vi "Read states.vi"(8 "error in (no error)":errorcluster, 11 "NewTestTactic in":refnum<class "NewTestTactic.lvclass">) -> (0 "error out":errorcluster, 2 "states":T1, 3 "NewTestTactic out":refnum<class "NewTestTactic.lvclass">)   [LabVIEW 2022 SP3, in "NewTestTactic.lvclass"]
uses:
  NewTestTactic.lvclass
  Control 1.ctl
  NewTestTactic.lvclass/NewTestTactic.ctl
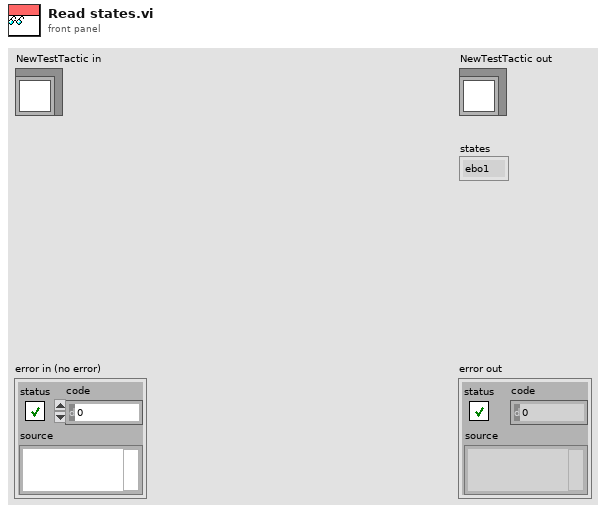
[diagram p1: front panel]
types:
  T1 = typedef "Control 1.ctl" = enum16{"ebo1", "ebo2", "bo3"}
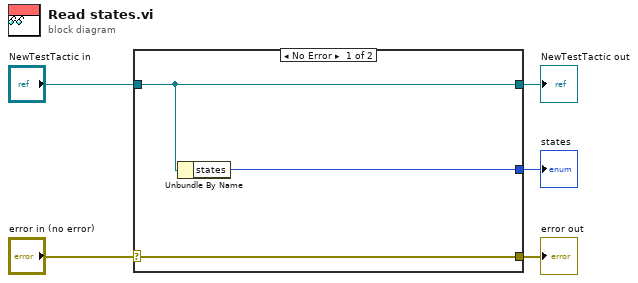
[diagram p0: block diagram]
diagram:
  n1 = case shown="No Error" "error in (no error)" {
    selector: "error in (no error)" -> [w8 w9]
    tunnel: [w8 w9] -> w4
    tunnel: [w7 w10] -> w2
    tunnel: "NewTestTactic in" -> [w7 w10]
    tunnel: [w6 _] -> w1
    frame No Error {
      n2 = Unbundle By Name(w7) -> ("states"=w6:T1)
    }
    frame Error {
    }
  }
  "error out" <- w4
  "NewTestTactic out" <- w2
  "states" <- w1
